vi "CaptureZSpan.vi"(8 "error in (no error)":errorcluster, 9 "Center Frequency (Hz)":dbl, 10 "Sweep Time (s)":dbl, 11 "SpecA_ESA in":refnum<class "SpecA_ESA.lvclass">) -> (0 "error out":errorcluster, 2 "Captured Waveform":waveform(dbl)(graph), 3 "SpecA_ESA out":refnum<class "SpecA_ESA.lvclass">)   [LabVIEW 2014, in "SpecA_ESA.lvclass"]
uses:
  SpecA_ESA.lvclass
  SpecA_ESA.lvclass/SpecA_ESA.ctl
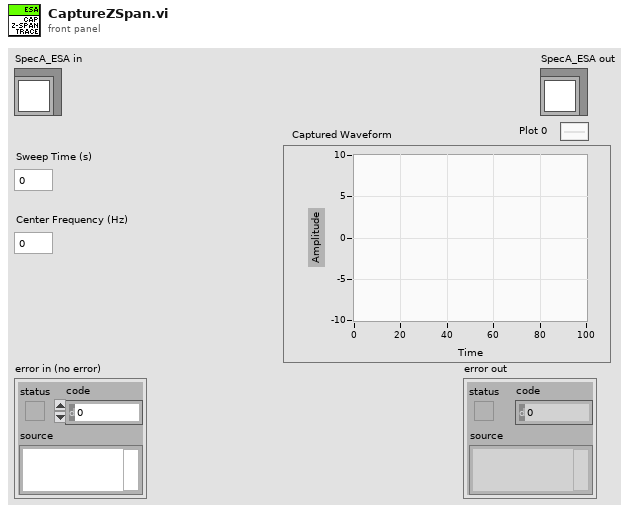
[diagram p1: front panel]
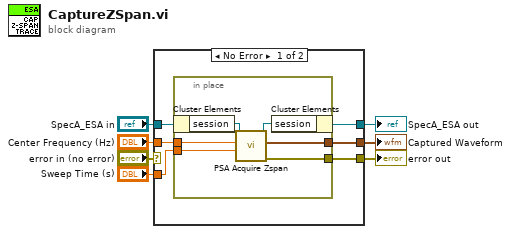
[diagram p0: block diagram]
diagram:
  n1 = case shown="No Error" "error in (no error)" {
    selector: "error in (no error)" -> [_ w21]
    tunnel: "SpecA_ESA in" -> [w13 w20]
    tunnel: [w12 _] -> w6
    tunnel: [w11 w20] -> w5
    tunnel: [w10 w21] -> w4
    tunnel: "Sweep Time (s)" -> [w9 _]
    tunnel: "Center Frequency (Hz)" -> [w8 _]
    frame No Error {
      n2 = in-place {
        in-place-border: [w17] -> w12
        in-place-border: [w16] -> w10
        in-place-border: w9 -> [w15]
        in-place-border: w8 -> [w14]
        n3 = in-place-cluster #1(w13) -> ("session"=w19:refnum<visa-resource-name>)
        n4 = call "PSA Acquire Zspan.vi"("Sweep Time (s)"=w15, "Center Frequency (Hz)"=w14, "VISA Refnum in"=w19) -> ("error out"=w16:errorcluster, "captured waveform"=w17:waveform(dbl), "VISA Refnum out"=w18:refnum<visa-resource-name>)  [unwired: 6 in]
        n5 = in-place-cluster #1("session"=w18) -> (w11:refnum<class "SpecA_ESA.lvclass">)
      }
    }
    frame Error {
    }
  }
  "error out" <- w4
  "SpecA_ESA out" <- w5
  "Captured Waveform" <- w6
